vi "Function_syringeSetting.vi"(2 "Direction":string, 3 "target volume- string":string, 5 "error in":errorcluster, 7 "VISA resource name in":refnum<visa-resource-name>, 8 "units":string, 9 "set rate- string":string, 10 "diameter(mm)-string":string, 11 "address (string)":string) -> (4 "error out":errorcluster, 6 "VISA resource name out":refnum<visa-resource-name>)   [LabVIEW 2020]
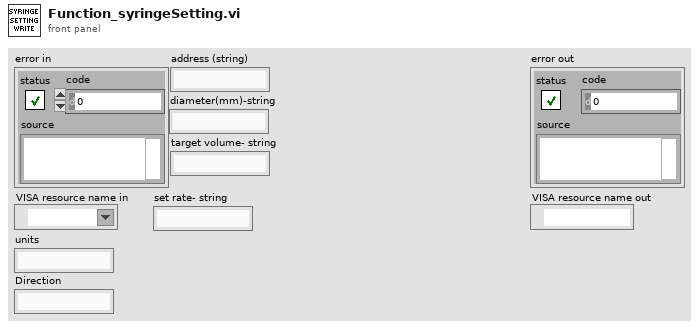
[diagram p1: front panel]
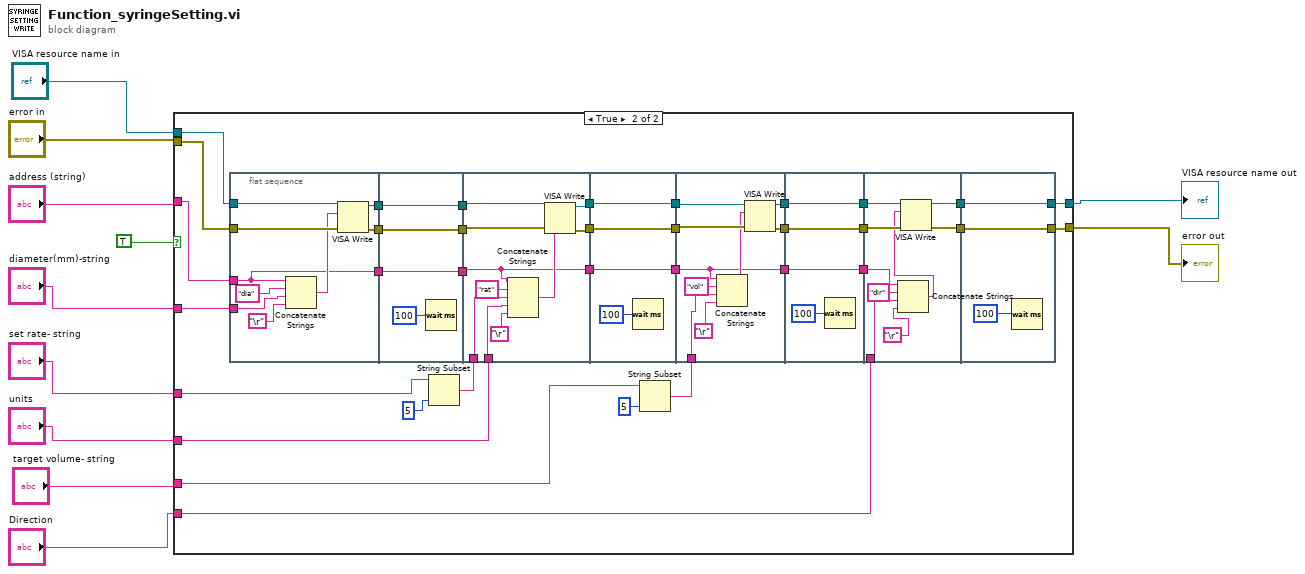
[diagram p0: block diagram]
diagram:
  n1 = case shown="True" TRUE {
    tunnel: "VISA resource name in" -> [w13 w47]
    tunnel: "error in" -> [w12 w46]
    tunnel: [w13 w45] -> w9
    tunnel: [w12 w44] -> w8
    tunnel: "address (string)" -> [_ w43]
    tunnel: "units" -> [_ w42]
    tunnel: "Direction" -> [_ w23]
    tunnel: "set rate- string" -> [_ w16]
    tunnel: "diameter(mm)-string" -> [_ w15]
    tunnel: "target volume- string" -> [_ w14]
    frame False {
    }
    frame True {
      n2 = flat-sequence {
        tunnel: w47 -> [w56]
        tunnel: w46 -> [w55]
        tunnel: [w54] -> w41
        tunnel: [w53] -> w39
        tunnel: w43 -> [w49]
        tunnel: [w49] -> w37
        tunnel: w15 -> [w48]
        tunnel: w41 -> [w60]
        tunnel: [w60] -> w40
        tunnel: w39 -> [w59]
        tunnel: [w59] -> w38
        tunnel: w37 -> [w58]
        tunnel: [w58] -> w36
        tunnel: w40 -> [w70]
        tunnel: w38 -> [w68]
        tunnel: w36 -> [w61]
        tunnel: w19 -> [w65]
        tunnel: w42 -> [w64]
        tunnel: [w69] -> w35
        tunnel: [w67] -> w33
        tunnel: [w61] -> w31
        tunnel: w35 -> [w74]
        tunnel: [w74] -> w34
        tunnel: w33 -> [w73]
        tunnel: [w73] -> w32
        tunnel: w31 -> [w72]
        tunnel: [w72] -> w30
        tunnel: w34 -> [w81]
        tunnel: w32 -> [w80]
        tunnel: w30 -> [w75]
        tunnel: w17 -> [w77]
        tunnel: [w82] -> w29
        tunnel: [w83] -> w28
        tunnel: [w75] -> w25
        tunnel: w29 -> [w87]
        tunnel: w28 -> [w86]
        tunnel: [w87] -> w27
        tunnel: [w86] -> w26
        tunnel: w25 -> [w84]
        tunnel: [w84] -> w24
        tunnel: w27 -> [w96]
        tunnel: w26 -> [w93]
        tunnel: w24 -> [w90]
        tunnel: w23 -> [w88]
        tunnel: [w95] -> w22
        tunnel: [w94] -> w21
        tunnel: [w98] -> w44
        tunnel: [w99] -> w45
        tunnel: w22 -> [w99]
        tunnel: w21 -> [w98]
        frame #0 {
          n3 = Concatenate Strings(w49, "dia" ("string"), w48, "\r") -> (w51:string)
          n4 = VISA Write(VISA resource name=w56, write buffer=w51, error in (no error)=w55) -> (VISA resource name out=w54:refnum<visa-resource-name>, error out=w53:errorcluster)  [unwired: 1 out]
        }
        frame #1 {
          n5 = Wait (ms)(milliseconds to wait=u32 100) -> ()  [unwired: 1 out]
        }
        frame #2 {
          n6 = Concatenate Strings(w61, "rat" ("string"), w65, w64, "\r") -> (w62:string)
          n7 = VISA Write(VISA resource name=w70, write buffer=w62, error in (no error)=w68) -> (VISA resource name out=w69:refnum<visa-resource-name>, error out=w67:errorcluster)  [unwired: 1 out]
        }
        frame #3 {
          n8 = Wait (ms)(milliseconds to wait=u32 100) -> ()  [unwired: 1 out]
        }
        frame #4 {
          n9 = Concatenate Strings(w75, "vol" ("string"), w77, "\r") -> (w76:string)
          n10 = VISA Write(VISA resource name=w81, write buffer=w76, error in (no error)=w80) -> (VISA resource name out=w82:refnum<visa-resource-name>, error out=w83:errorcluster)  [unwired: 1 out]
        }
        frame #5 {
          n11 = Wait (ms)(milliseconds to wait=u32 100) -> ()  [unwired: 1 out]
        }
        frame #6 {
          n12 = Concatenate Strings(w90, "dir" ("string"), w88, "\r") -> (w92:string)
          n13 = VISA Write(VISA resource name=w96, write buffer=w92, error in (no error)=w93) -> (VISA resource name out=w95:refnum<visa-resource-name>, error out=w94:errorcluster)  [unwired: 1 out]
        }
        frame #7 {
          n14 = Wait (ms)(milliseconds to wait=u32 100) -> ()  [unwired: 1 out]
        }
      }
      n15 = String Subset(string=w16, length (rest)=5 ("length (rest)")) -> (substring=w19:string)  [unwired: 1 in]
      n16 = String Subset(string=w14, length (rest)=5 ("length (rest)")) -> (substring=w17:string)  [unwired: 1 in]
    }
  }
  "error out" <- w8
  "VISA resource name out" <- w9
